vi "SineOrSawtoothInverse.vi"(3 "error in (no error)":errorcluster, 4 "Parameters":T2={"number of planes"=4, "z step"=1.9999999999999998e-05, "pixel dwell time"=1.0000000000000001e-11, "z frequency"=10.0, "number of pixels"=100, "smooth points"=10, "smooth line"=10, "Sine\nSawtooth"=FALSE, "PointSorting"=0, "Sort Points"=FALSE, "X-pixels"=256.0, "Y-lines"=256.0, "pixelstoµm"=256.0, "zoom"=1.0, "Time offset"=1.0000000000000001e-11} {"zoom" min=0.5 step=0.1; "Y-lines" min=1 step=1; "X-pixels" min=1 step=1; "PointSorting" items=["No Difference", "Every Second Point", "Down / Up"]; "smooth line" min=1; "smooth points" min=1; "number of pixels" min=1; "z frequency" format="%_4g"; "number of planes" min=1}, 5 "DutyCluster":T1 {"Iteration" items=["first iteration", "second iteration"]}) -> (0 "error out":errorcluster, 1 "DutyCluster":T1 {"Iteration" items=["first iteration", "second iteration"]})   [LabVIEW 2010]
uses:
  TypeDefs/DutyCluster.ctl
  TypeDefs/ParameterCluster.ctl
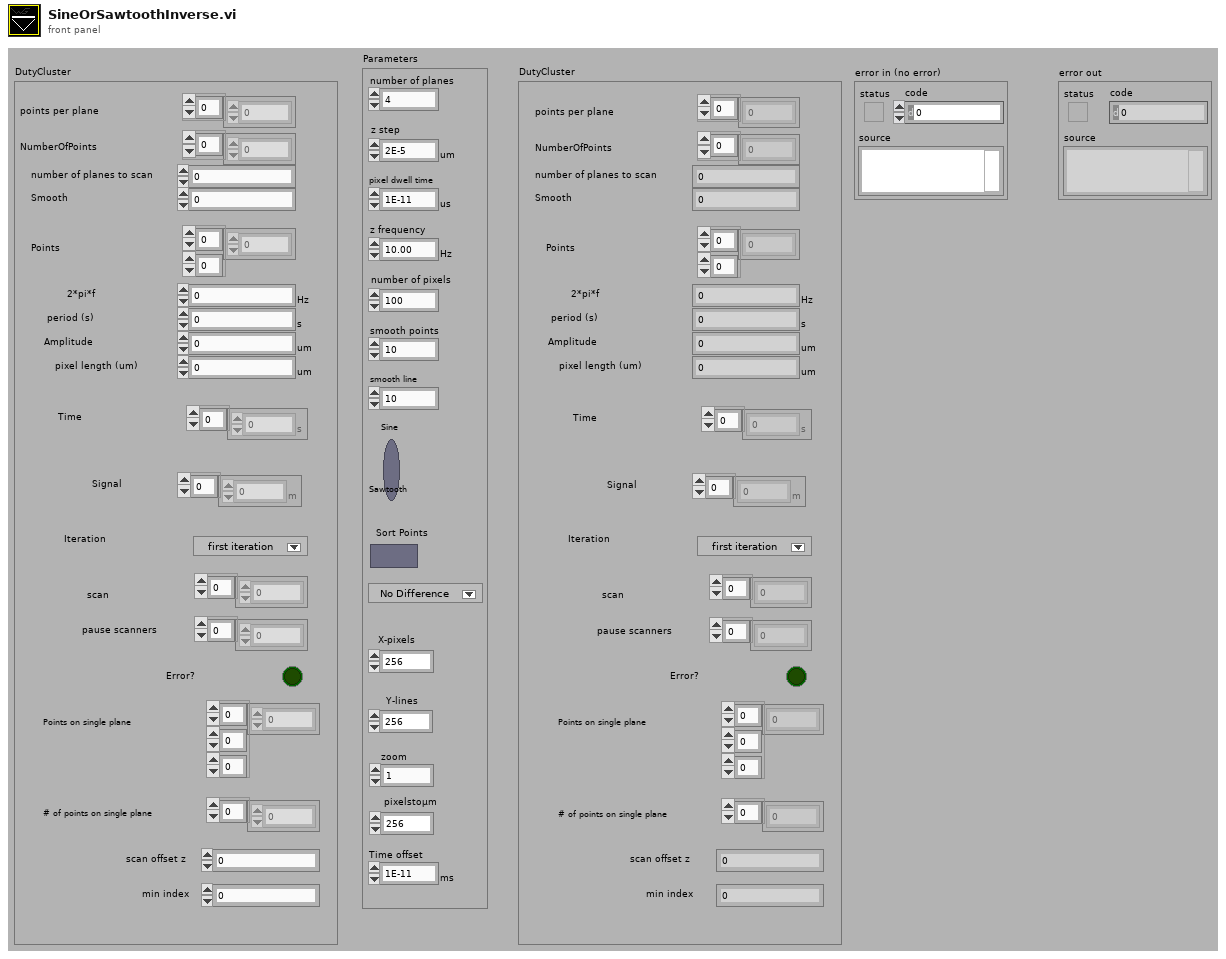
[diagram p1: front panel]
types:
  T1 = typedef "DutyCluster.ctl" = cluster{"points per plane":i32[], "NumberOfPoints":i32[], "number of planes to scan":i32, "Smooth":i32, "Points":dbl[][], "2*pi*f":dbl[unit], "period (s)":dbl[unit], "Amplitude":dbl[unit], "pixel length (um)":dbl[unit], "Time":dbl[unit][], "Signal":dbl[unit][], "Iteration":u16, "scan":i32[], "pause scanners":i32[], "Error?":bool, "Points on single plane":dbl[][][], "# of points on single plane":i32[], "scan offset z":i32, "min index":i32}
  T2 = typedef "ParameterCluster.ctl" = cluster{"number of planes":i32, "z step":dbl[unit], "pixel dwell time":dbl[unit], "z frequency":dbl[unit], "number of pixels":i32, "smooth points":i32, "smooth line":i32, "Sine\nSawtooth":bool, "PointSorting":u16, "Sort Points":bool, "X-pixels":sgl, "Y-lines":sgl, "pixelstoµm":dbl, "zoom":dbl, "Time offset":dbl[unit]}
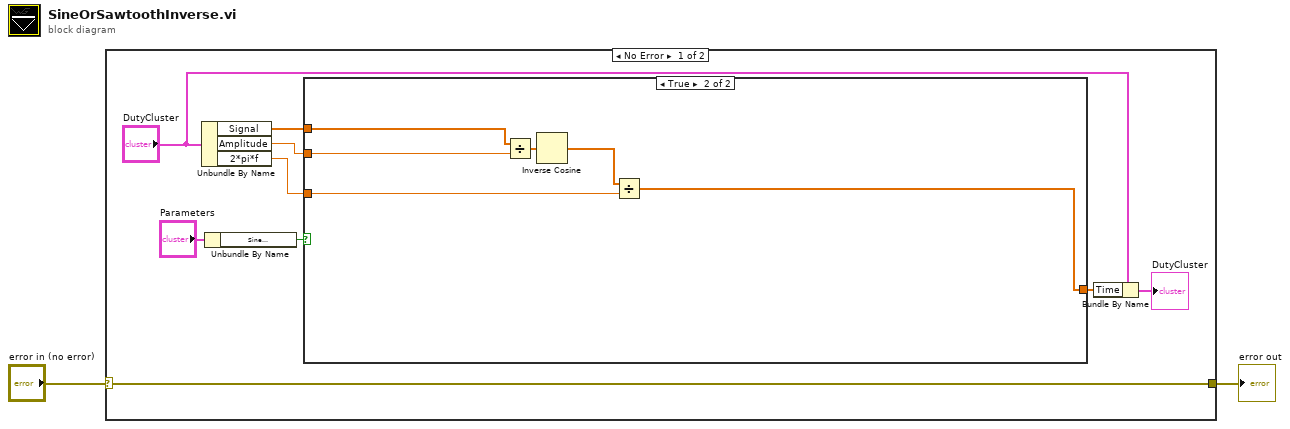
[diagram p0: block diagram]
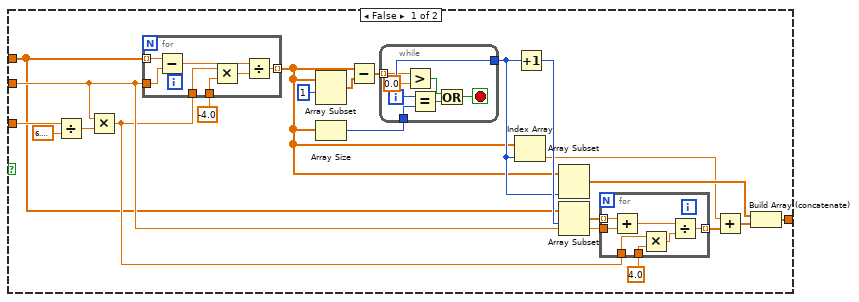
[diagram p2: hidden frame]
diagram:
  n1 = case shown="No Error" "error in (no error)" {
    selector: "error in (no error)" -> [w3 w60]
    tunnel: [w3 w60] -> w1
    frame No Error {
      n2 = Unbundle By Name("DutyCluster") -> ("Signal"=w11:dbl[unit][], "Amplitude"=w10:dbl[unit], "2*pi*f"=w9:dbl[unit])
      n3 = Unbundle By Name("Parameters") -> ("Sine\nSawtooth"=w7:bool)
      n4 = case shown="True" w7 {
        tunnel: w9 -> [w31 w55]
        tunnel: w10 -> [w23 w57]
        tunnel: w11 -> [w16 w58]
        tunnel: [w12 w54] -> w4
        frame False {
          n5 = Divide(x=w31, y=6.283185307179586) -> (x/y=w30:dbl[unit])
          n6 = Multiply(x=w23, y=w30) -> (x*y=w22:dbl[unit])
          n7 = for {
            tunnel: w16 -> [w53] mode=indexing
            tunnel: w22 -> [w49]
            tunnel: [w51] -> w15 mode=indexing
            tunnel: -4.0 ("value") -> [w50]
            tunnel: w23 -> [w47]
            n8 = Subtract(x=w53, y=w47) -> (x-y=w52:dbl[unit])
            n9 = Multiply(x=w49, y=w50) -> (x*y=w48:dbl[unit])
            n10 = Divide(x=w52, y=w48) -> (x/y=w51:dbl[unit])
          }
          n11 = Array Subset(array=w15, index=1) -> (w27:dbl[unit][])  [unwired: 1 in]
          n12 = Array Size(array=w15) -> (size(s)=w14:i32)
          n13 = Subtract(x=w15, y=w27) -> (x-y=w26:dbl[unit][])
          n14 = while {
            tunnel: w26 -> [w42] mode=indexing
            tunnel: [w46] -> w19
            tunnel: w14 -> [w45]
            i -> [w46]
            stop <- w43 stop-if-true
            n15 = Greater?(x=w42, y=dbl[unit] 0.0) -> (0:w40:bool)
            n16 = Equal?(x=w46, y=w45) -> (x = y?=w44:bool)
            n17 = Or(x=w40, y=w44) -> (x .or. y?=w43:bool)
          }
          n18 = Index Array(array=w15, index=w19) -> (element=w18:dbl[unit])
          n19 = Increment(x=w19) -> (x+1=w25:i32)
          n20 = Array Subset(array=w15, length=w19) -> (w20:dbl[unit][])  [unwired: 1 in]
          n21 = Array Subset(array=w16, index=w25) -> (w24:dbl[unit][])  [unwired: 1 in]
          n22 = for {
            tunnel: w22 -> [w36]
            tunnel: [w38] -> w17 mode=indexing
            tunnel: 4.0 ("value") -> [w37]
            tunnel: w23 -> [w34]
            tunnel: w24 -> [w33] mode=indexing
            n23 = Add(x=w33, y=w34) -> (x+y=w39:dbl[unit])
            n24 = Multiply(x=w36, y=w37) -> (x*y=w35:dbl[unit])
            n25 = Divide(x=w39, y=w35) -> (x/y=w38:dbl[unit])
          }
          n26 = Add(x=w18, y=w17) -> (x+y=w13:dbl[unit][])
          n27 = Build Array (concatenate)(w20, w13) -> (w12:dbl[unit][])
        }
        frame True {
          n28 = Divide(x=w58, y=w57) -> (x/y=w59:dbl[])
          n29 = Inverse Cosine(1:w59) -> (0:w56:dbl[])
          n30 = Divide(x=w56, y=w55) -> (x/y=w54:dbl[unit][])
        }
      }
      n31 = Bundle By Name(cluster="DutyCluster", "Time"=w4) -> (→"DutyCluster":T1)
    }
    frame Error {
    }
  }
  "error out" <- w1
